vi "Get SysDef Root Node ID (SubVI).vi"(8 "error in (no error)":errorcluster, 11 "SysDef Refnum In":refnum<k39>) -> (0 "error out":errorcluster, 2 "Root NodeID Out":u64, 3 "SysDef Refnum Out":refnum<k39>)   [LabVIEW 2026, in "FPGA Addon Test Class.lvclass"]
uses:
  FPGA Addon Test Class.lvclass
  C:/Users/Administrator/Desktop/Jatin/All DNC DLLs/NationalInstruments.VeriStand.SystemDefinitionAPI.dll
  Jatin/All DNC DLLs/NationalInstruments.VeriStand.SystemDefinitionAPI.dll
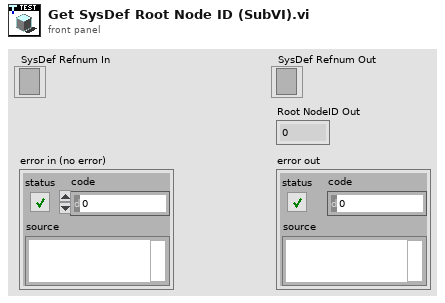
[diagram p1: front panel]
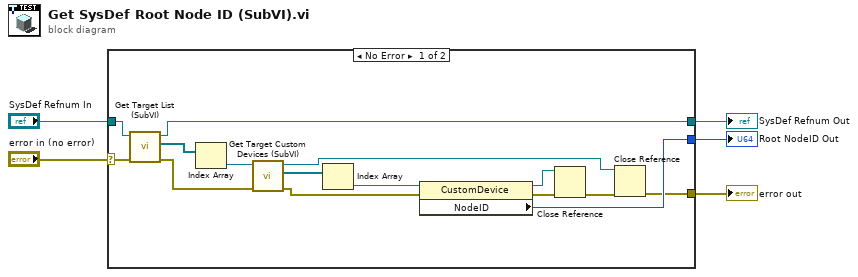
[diagram p0: block diagram]
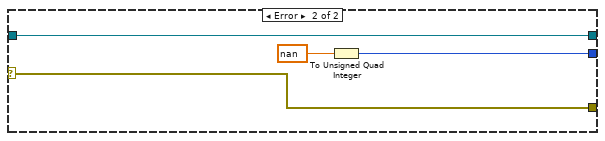
[diagram p2: hidden frame]
diagram:
  n1 = case shown="No Error" "error in (no error)" {
    selector: "error in (no error)" -> [w13 w24]
    tunnel: [w7 w24] -> w5
    tunnel: "SysDef Refnum In" -> [w14 w21]
    tunnel: [w12 w22] -> w2
    tunnel: [w11 w21] -> w1
    frame No Error {
      n2 = call "Get Target List (SubVI).vi"("error in (no error)"=w13, "NationalInstruments.VeriStand.SystemDefinitionAPI.SystemDefinition"=w14) -> ("error out"=w19:errorcluster, "Target List Refnums"=w15:refnum<k39>[], "NationalInstruments.VeriStand.SystemDefinitionAPI.SystemDefinition"=w11:refnum<k39>)  [unwired: 7 in]
      n3 = Index Array(array=w15) -> (element=w16:refnum<k39>)  [unwired: 1 in]
      n4 = call "Get Target Custom Devices (SubVI).vi"("error in (no error)"=w19, "NationalInstruments.VeriStand.SystemDefinitionAPI.Target"=w16) -> ("error out"=w20:errorcluster, "Custom Devices Refnums"=w17:refnum<k39>[], "NationalInstruments.VeriStand.SystemDefinitionAPI.Target"=w6:refnum<k39>)  [unwired: 6 in, 1 out]
      n5 = Index Array(array=w17) -> (element=w18:refnum<k39>)  [unwired: 1 in]
      n6 = property class="CustomDevice"(reference=w18, error in=w20) -> (reference out=w9:refnum<k39>, error out=w10:errorcluster, "NodeID"=w12:u64)
      n7 = Close Reference(reference=w9, error in (no error)=w10) -> (error out=w8:errorcluster)
      n8 = Close Reference(reference=w6, error in (no error)=w8) -> (error out=w7:errorcluster)
    }
    frame Error {
      n9 = To Unsigned Quad Integer(1:nan) -> (0:w22:u64)
    }
  }
  "error out" <- w5
  "Root NodeID Out" <- w2
  "SysDef Refnum Out" <- w1
